vi "Path to String.vi"(1 "Path":path) -> (0 "Path String":string)   [LabVIEW 2020, in "feature_detection.lvlib" / "DNN Detection Model.lvclass"]
uses:
  DNN Detection Model.lvclass
  DNN Detection Model.lvclass/DNN Detection Model.ctl
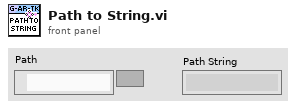
[diagram p1: front panel]
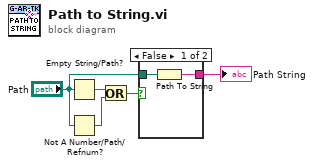
[diagram p0: block diagram]
diagram:
  n1 = Empty String/Path?(string/path="Path") -> (empty?=w4:bool)
  n2 = Not A Number/Path/Refnum?(number/path/refnum="Path") -> (NaN/Path/Refnum?=w3:bool)
  n3 = Or(x=w4, y=w3) -> (x .or. y?=w2:bool)
  n4 = case shown="False" w2 {
    tunnel: "Path" -> [w7 _]
    tunnel: [w6 _] -> w1
    frame False {
      n5 = Path To String(path=w7) -> (string=w6:string)
    }
    frame True {
    }
  }
  "Path String" <- w1
